vi "Create Error Qs.vi"(8 "error in (no error)":errorcluster) -> (0 "error out":errorcluster, 3 "Error Qs":T1, 5 "Error Publishing Q":refnum<queue>)   [LabVIEW 2011, in "AIT 1553 Custom Device.lvlib"]
uses:
  AIT 1553 Custom Device.lvlib
  RT Controls/Error Qs.ctl
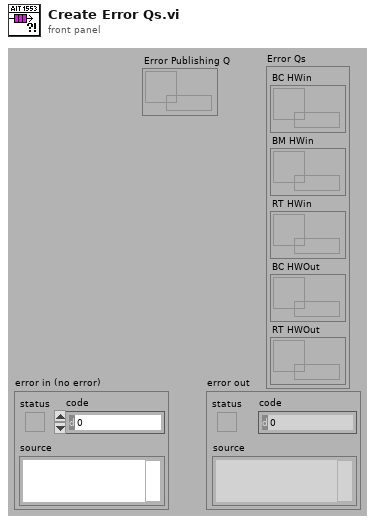
[diagram p1: front panel]
types:
  T1 = typedef "AIT 1553 Custom Device.lvlib/Error Qs.ctl" = cluster{"BC HWin":refnum<queue>, "BM HWin":refnum<queue>, "RT HWin":refnum<queue>, "BC HWOut":refnum<queue>, "RT HWOut":refnum<queue>}
  T2 = cluster{"[0]":refnum<queue>, "[1]":refnum<queue>, "[2]":refnum<queue>, "[3]":refnum<queue>, "[4]":refnum<queue>}
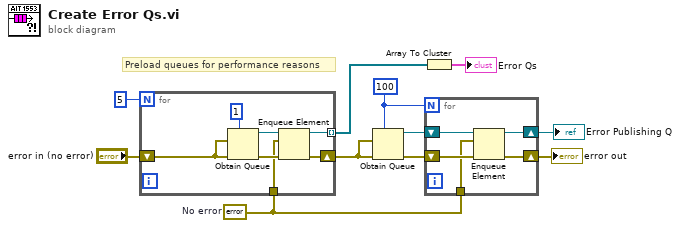
[diagram p0: block diagram]
diagram:
  w2 = errorcluster {"status"=FALSE, "code"=0, "source"=""}  # No error
  w1 = 100 ("max queue size (-1, unlimited)")
  # "Preload queues for performance reasons"
  n1 = for {
    N: 5 -> [_]
    shift-right: [w14] -> w7
    shift-left: "error in (no error)" -> [w18]
    tunnel: [w15] -> w9 mode=indexing
    tunnel: w2 -> [w12]
    n2 = Obtain Queue(max queue size (-1, unlimited)=1, element data type=w18, error in (no error)=w18) -> (queue out=w16:refnum<queue>, error out=w13:errorcluster)  [unwired: 2 in, 1 out]
    n3 = Enqueue Element(queue=w16, element=w12, error in (no error)=w13) -> (queue out=w15:refnum<queue>, error out=w14:errorcluster)  [unwired: 1 in, 1 out]
  }
  n4 = Obtain Queue(max queue size (-1, unlimited)=w1, element data type=w7, error in (no error)=w7) -> (queue out=w5:refnum<queue>, error out=w6:errorcluster)  [unwired: 2 in, 1 out]
  n5 = Array To Cluster(array=w9) -> (cluster=→"Error Qs":T2)
  n6 = for {
    N: w1 -> [_]
    shift-right: [w20] -> w3
    shift-left: w6 -> [w23]
    shift-right: [w21] -> w4
    shift-left: w5 -> [w22]
    tunnel: w2 -> [w19]
    n7 = Enqueue Element(queue=w22, element=w19, error in (no error)=w23) -> (queue out=w21:refnum<queue>, error out=w20:errorcluster)  [unwired: 1 in, 1 out]
  }
  "error out" <- w3
  "Error Publishing Q" <- w4
